vi "Read Topologies.vi"(8 "error in (no error)":errorcluster, 11 "SLSC Switch in":refnum<class "SLSC Switch.lvclass">) -> (0 "error out":errorcluster, 2 "Topologies":T1[](array[typedef]), 3 "SLSC Switch out":refnum<class "SLSC Switch.lvclass">)   [LabVIEW 2015, in "SLSC Switch.lvlib" / "SLSC Switch.lvclass"]
uses:
  SLSC Switch.lvclass
  Controls/Topology.ctl
  Controls/JSON.InitialState.ctl
  Controls/MuxList Entry.ctl
  SLSC Switch.lvclass/SLSC Switch.ctl
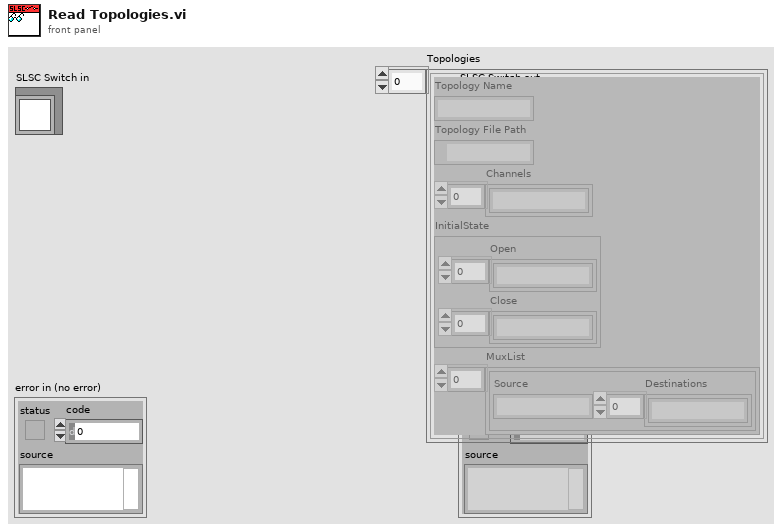
[diagram p1: front panel]
types:
  T1 = typedef "SLSC Switch.lvlib/SLSC Switch.lvclass/Topology.ctl" = cluster{"Topology Name":string, "Topology File Path":path, "Channels":string[], "InitialState":T2, "MuxList":T3[]}
  T2 = typedef "SLSC Switch.lvlib/SLSC Switch.lvclass/JSON.InitialState.ctl" = cluster{"Open":string[], "Close":string[]}
  T3 = typedef "SLSC Switch.lvlib/SLSC Switch.lvclass/MuxList Entry.ctl" = cluster{"Source":string, "Destinations":string[]}
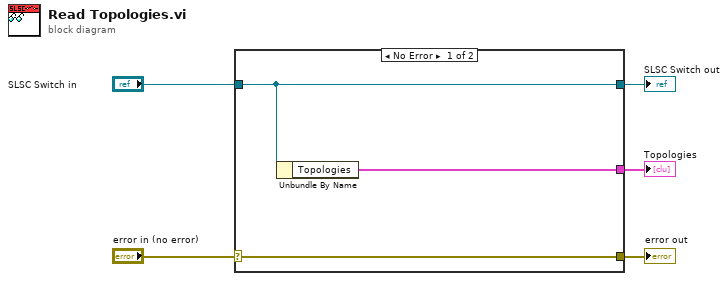
[diagram p0: block diagram]
diagram:
  n1 = case shown="No Error" "error in (no error)" {
    selector: "error in (no error)" -> [w8 w9]
    tunnel: [w8 w9] -> w4
    tunnel: [w7 w10] -> w2
    tunnel: "SLSC Switch in" -> [w7 w10]
    tunnel: [w6 _] -> w1
    frame No Error {
      n2 = Unbundle By Name(w7) -> ("Topologies"=w6:T1[])
    }
    frame Error {
    }
  }
  "error out" <- w4
  "SLSC Switch out" <- w2
  "Topologies" <- w1
